vi "UILoadDefaults.vi"   [LabVIEW 2014, in "UILib.lvlib"]
uses:
  UILib.lvlib
  <vilib>/Rock Robotics/WPI/Solenoid/WPI_SolenoidValue.ctl
  <vilib>/Utility/config.llb/Read Key (Double).vi
  <vilib>/Utility/config.llb/Read Key (String).vi
  <vilib>/Utility/config.llb/NI_LVConfig.lvlib
types:
  T1 = typedef "WPI_SolenoidValue.ctl" = enum16{"Off", "On", "Forward", "Reverse"}
  T2 = typedef "NI_LVConfig.lvlib/Config Data RefNum.ctl" = refnum<k1>
  T3 = enum16{"open", "replace", "create", "open or create", "replace or create", "replace or create with confirmation"}
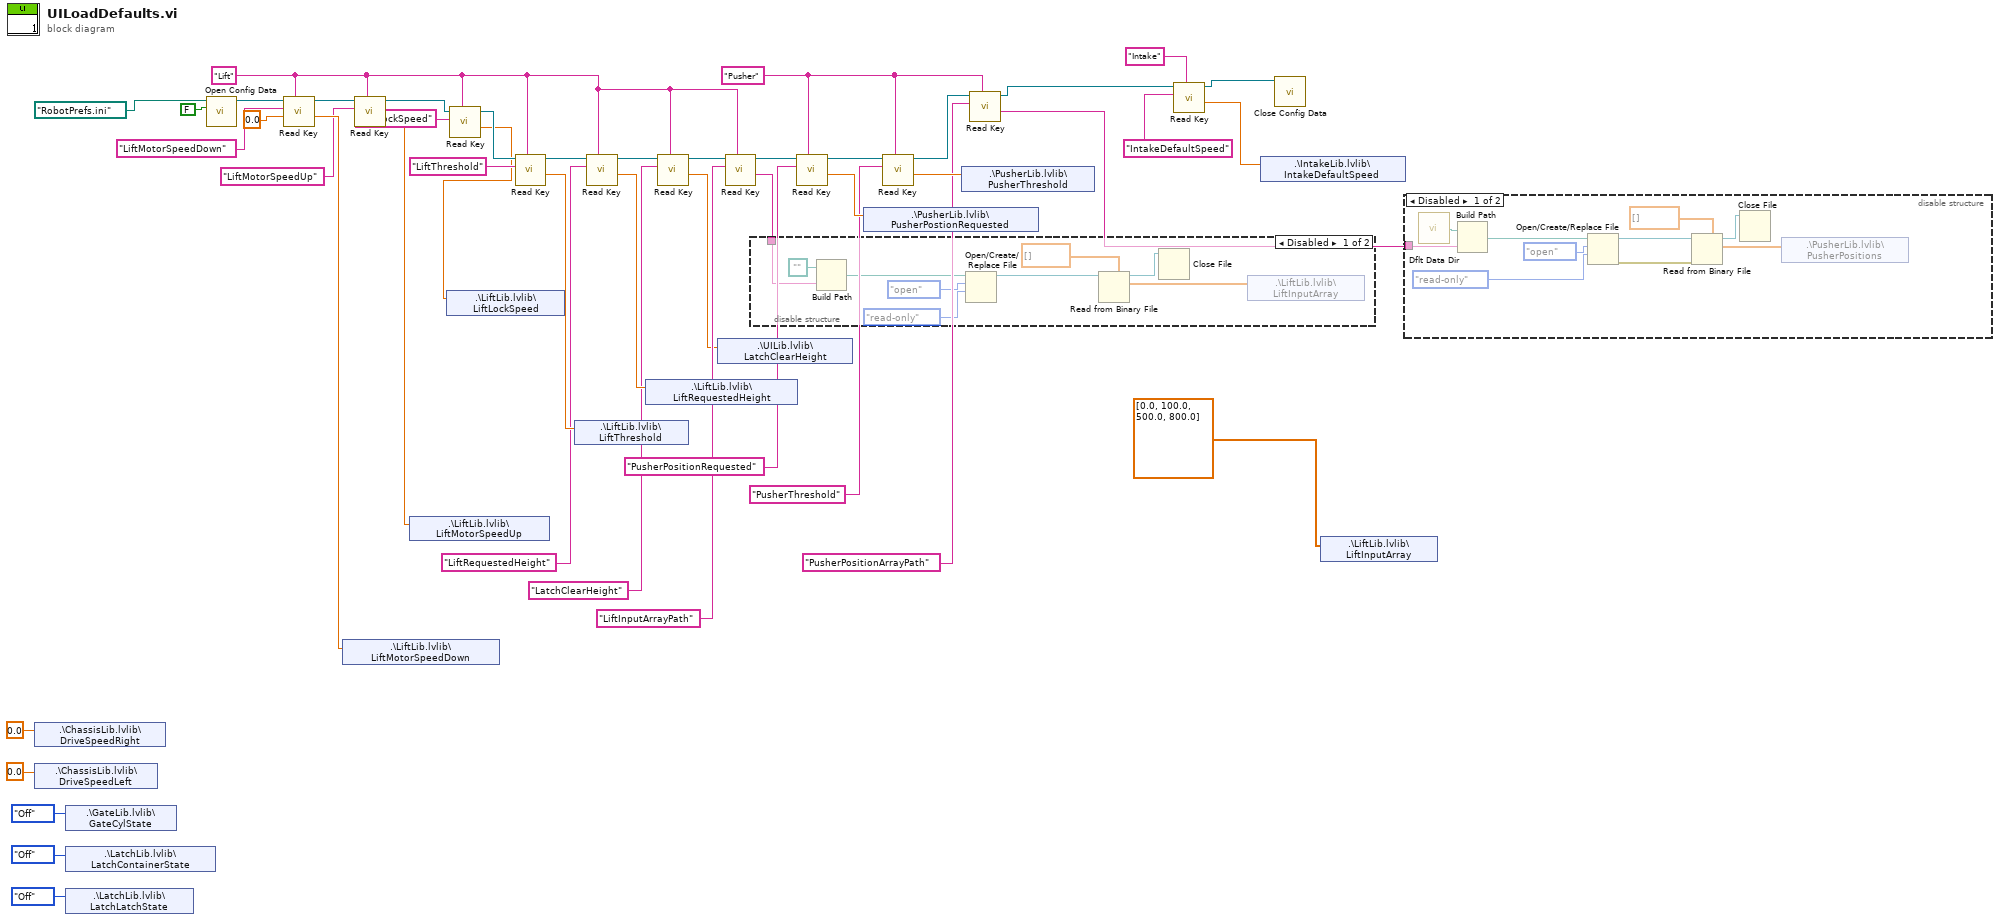
[diagram p0: block diagram]
diagram:
  w22 = "Pusher" ("section")
  w3 = "Lift" ("section")
  n1 = shared-variable ".\\ChassisLib.lvlib\\DriveSpeedRight"(0.0 ("DriveSpeedRight")) -> ()  [unwired: 1 in, 1 out]
  n2 = shared-variable ".\\ChassisLib.lvlib\\DriveSpeedLeft"(0.0 ("DriveSpeedLeft")) -> ()  [unwired: 1 in, 1 out]
  n3 = shared-variable ".\\GateLib.lvlib\\GateCylState"(WPI_SolenoidValue."Off" ("GateCylState")) -> ()  [unwired: 1 in, 1 out]
  n4 = shared-variable ".\\LatchLib.lvlib\\LatchContainerState"(WPI_SolenoidValue."Off" ("LatchContainerState")) -> ()  [unwired: 1 in, 1 out]
  n5 = shared-variable ".\\LatchLib.lvlib\\LatchLatchState"(WPI_SolenoidValue."Off" ("LatchLatchState")) -> ()  [unwired: 1 in, 1 out]
  n6 = call <vilib>:"Open Config Data.vi"("create file if necessary (T)"=FALSE, "configuration file path"=path "/RobotPrefs.ini") -> ("refnum"=w43:T2)  [unwired: 7 in, 2 out]
  n7 = call-poly <vilib>:"Read Key.vi"("section"=w3, "default value"=0.0, "key"="LiftMotorSpeedDown", "refnum"=w43) -> ("value"=w42:dbl, "refnum out"=w20:T2)  [unwired: 4 in, 2 out]
  n8 = shared-variable ".\\LiftLib.lvlib\\LiftMotorSpeedDown"(w42) -> ()  [unwired: 1 in, 1 out]
  n9 = call-poly <vilib>:"Read Key.vi"("section"=w3, "key"="LiftMotorSpeedUp", "refnum"=w20) -> ("value"=w39:dbl, "refnum out"=w5:T2)  [unwired: 5 in, 2 out]
  n10 = shared-variable ".\\LiftLib.lvlib\\LiftMotorSpeedUp"(w39) -> ()  [unwired: 1 in, 1 out]
  n11 = call-poly <vilib>:"Read Key.vi"("section"=w3, "key"="LiftLockSpeed", "refnum"=w5) -> ("value"=w1:dbl, "refnum out"=w4:T2)  [unwired: 5 in, 2 out]
  n12 = shared-variable ".\\LiftLib.lvlib\\LiftLockSpeed"(w1) -> ()  [unwired: 1 in, 1 out]
  n13 = call-poly <vilib>:"Read Key.vi"("section"=w3, "key"="LiftThreshold", "refnum"=w4) -> ("value"=w37:dbl, "refnum out"=w35:T2)  [unwired: 5 in, 2 out]
  n14 = shared-variable ".\\LiftLib.lvlib\\LiftThreshold"(w37) -> ()  [unwired: 1 in, 1 out]
  n15 = call-poly <vilib>:"Read Key.vi"("section"=w3, "key"="LiftRequestedHeight", "refnum"=w35) -> ("value"=w25:dbl, "refnum out"=w16:T2)  [unwired: 5 in, 2 out]
  n16 = shared-variable ".\\LiftLib.lvlib\\LiftRequestedHeight"(w25) -> ()  [unwired: 1 in, 1 out]
  n17 = call-poly <vilib>:"Read Key.vi"("section"=w3, "key"="LatchClearHeight", "refnum"=w16) -> ("value"=w13:dbl, "refnum out"=w15:T2)  [unwired: 5 in, 2 out]
  n18 = shared-variable ".\\UILib.lvlib\\LatchClearHeight"(w13) -> ()  [unwired: 1 in, 1 out]
  n19 = call-poly <vilib>:"Read Key.vi"("section"=w3, "key"="LiftInputArrayPath", "refnum"=w15) -> ("value"=w17:string, "refnum out"=w19:T2)  [unwired: 5 in, 2 out]
  n20 = disable-structure shown="Disabled" {
    disable-tunnel: w17 -> [w49 _]
    frame Disabled {
      n21 = Build Path(base path=path "", name or relative path=w49) -> (appended path=w48:path)
      n22 = Open/Create/Replace File(file path (use dialog)=w48, operation (0:open)=T3."open", access (0:read/write)=enum16{"read/write", "read-only", "write-only"}."read-only") -> (refnum out=w53:refnum<file>)  [unwired: 3 in, 2 out]
      n23 = Read from Binary File(5:dbl[] [], 11:w53) -> (2:w51:dbl[], 3:w50:refnum<file>)  [unwired: 4 in, 2 out]
      n24 = Close File(refnum=w50) -> ()  [unwired: 1 in, 2 out]
      n25 = shared-variable ".\\LiftLib.lvlib\\LiftInputArray"(w51) -> ()  [unwired: 1 in, 1 out]
    }
    frame Enabled {
    }
  }
  n26 = call-poly <vilib>:"Read Key.vi"("section"=w22, "key"="PusherPositionRequested", "refnum"=w19) -> ("value"=w32:dbl, "refnum out"=w31:T2)  [unwired: 5 in, 2 out]
  n27 = shared-variable ".\\PusherLib.lvlib\\PusherPostionRequested"(w32) -> ()  [unwired: 1 in, 1 out]
  n28 = call-poly <vilib>:"Read Key.vi"("section"=w22, "key"="PusherThreshold", "refnum"=w31) -> ("value"=w30:dbl, "refnum out"=w23:T2)  [unwired: 5 in, 2 out]
  n29 = shared-variable ".\\PusherLib.lvlib\\PusherThreshold"(w30) -> ()  [unwired: 1 in, 1 out]
  n30 = call-poly <vilib>:"Read Key.vi"("section"=w22, "key"="PusherPositionArrayPath", "refnum"=w23) -> ("value"=w18:string, "refnum out"=w12:T2)  [unwired: 5 in, 2 out]
  n31 = call-poly <vilib>:"Read Key.vi"("section"="Intake", "key"="IntakeDefaultSpeed", "refnum"=w12) -> ("value"=w10:dbl, "refnum out"=w11:T2)  [unwired: 5 in, 2 out]
  n32 = shared-variable ".\\IntakeLib.lvlib\\IntakeDefaultSpeed"(w10) -> ()  [unwired: 1 in, 1 out]
  n33 = call <vilib>:"Close Config Data.vi"("refnum"=w11) -> ()  [unwired: 9 in, 2 out]
  n34 = shared-variable ".\\LiftLib.lvlib\\LiftInputArray"(dbl[] [0.0, 100.0, 500.0, 800.0]) -> ()  [unwired: 1 in, 1 out]
  n35 = disable-structure shown="Disabled" {
    disable-tunnel: w18 -> [w57 _]
    frame Disabled {
      n36 = call <vilib>:"Dflt Data Dir.vi"() -> ("App:Default Data Directory"=w58:path)
      n37 = Build Path(base path=w58, name or relative path=w57) -> (appended path=w56:path)
      n38 = Open/Create/Replace File(file path (use dialog)=w56, operation (0:open)=T3."open", access (0:read/write)=enum16{"read/write", "read-only", "write-only"}."read-only") -> (refnum out=w62:refnum<file>, error out=w63:errorcluster)  [unwired: 3 in, 1 out]
      n39 = Read from Binary File(5:dbl[] [], 8:w63, 11:w62) -> (2:w59:dbl[], 3:w61:refnum<file>)  [unwired: 3 in, 2 out]
      n40 = Close File(refnum=w61) -> ()  [unwired: 1 in, 2 out]
      n41 = shared-variable ".\\PusherLib.lvlib\\PusherPositions"(w59) -> ()  [unwired: 1 in, 1 out]
    }
    frame Enabled {
    }
  }
